vi "Stage 3.3 Placing Process into subVIs.vi"() -> ()   [LabVIEW 2020]
uses:
  HRM-User_events.ctl
  HRM-init_cluster.ctl
panel:
  out "Process Error":errorcluster
  out "error out":errorcluster
  out "raw data":waveform(dbl)
  out "error out Hardware":errorcluster
  in  "Addition signal to remove (0) [s]":dbl
  out "Pulse":dbl
  out "Filtered":waveform(dbl)(graph)
  in  "Samples size (10) [s]":i32=10
  out "unfiltered wf":waveform(dbl)(graph)
  in  "Stop":bool
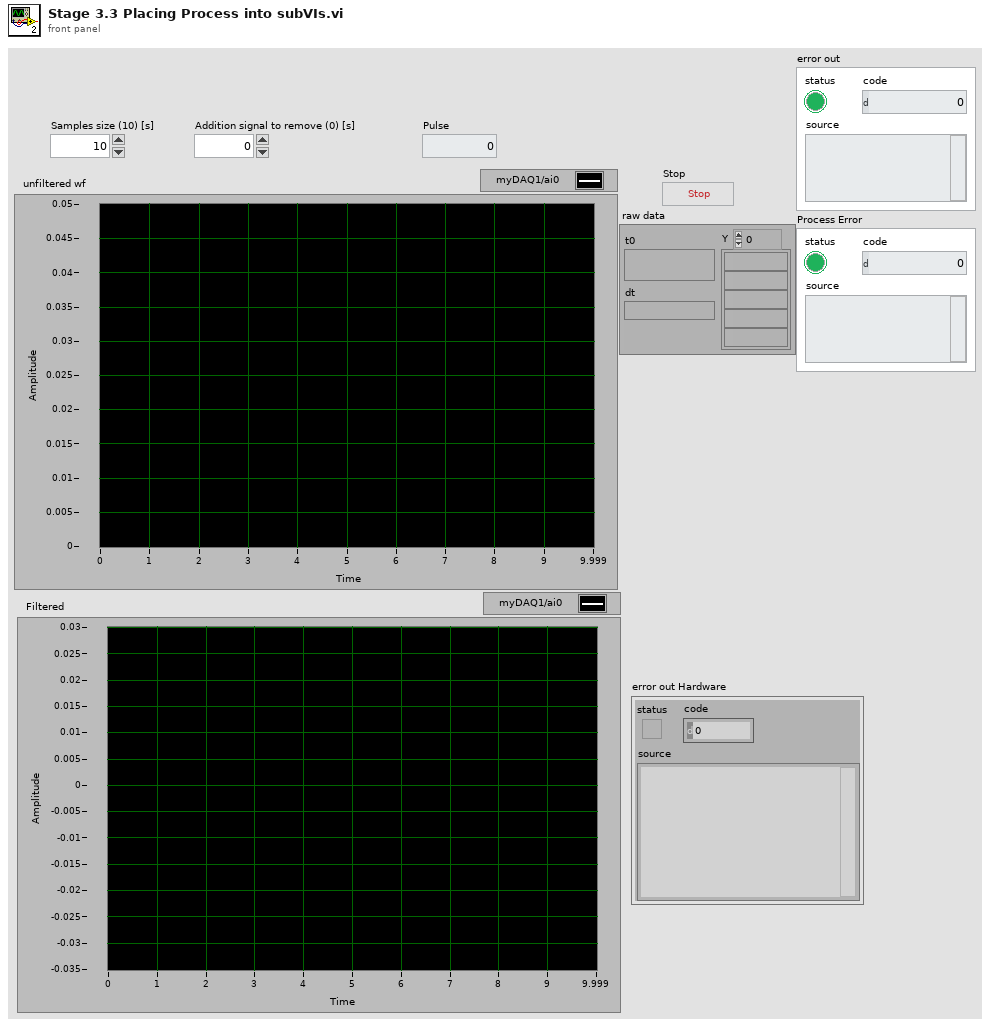
[diagram p1: front panel]
types:
  T1 = typedef "HRM-init_cluster.ctl" = cluster{"User events":T2}
  T2 = typedef "HRM-User_events.ctl" = cluster{"Signal to remove":refnum<user-event>, "Sample size":refnum<user-event>, "Filtered wf":refnum<user-event>, "Unfiltered wf":refnum<user-event>, "Raw wf":refnum<user-event>, "Pulse":refnum<user-event>, "stop":refnum<user-event>}
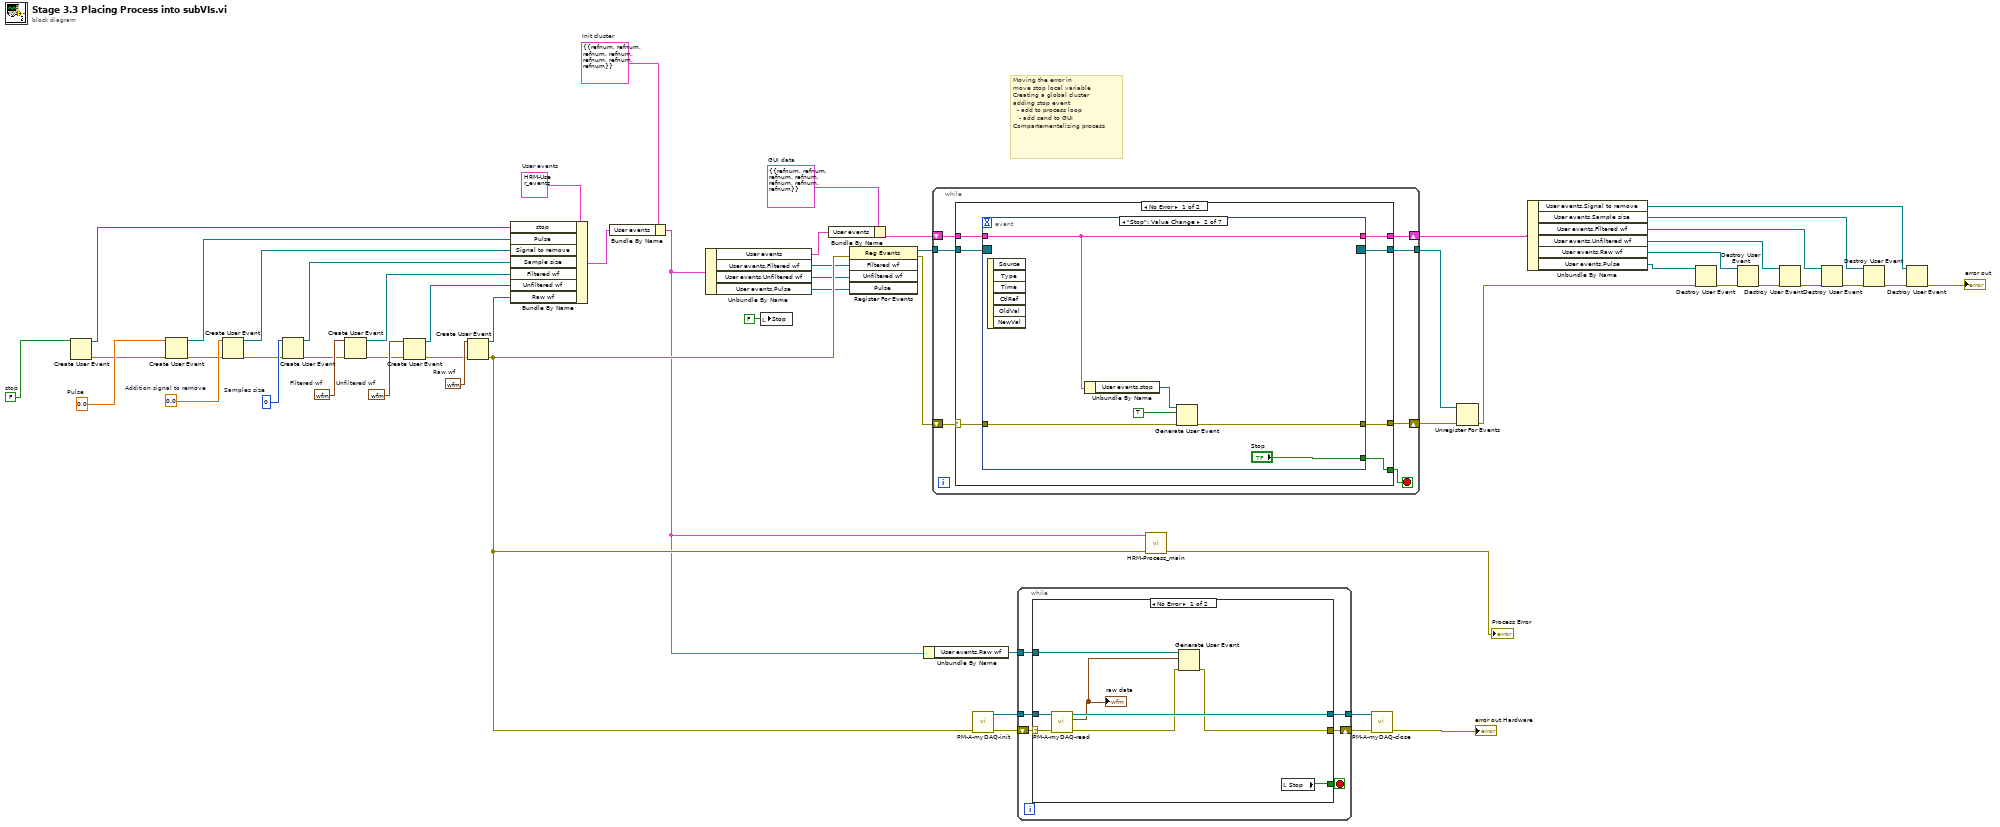
[diagram p0: block diagram]
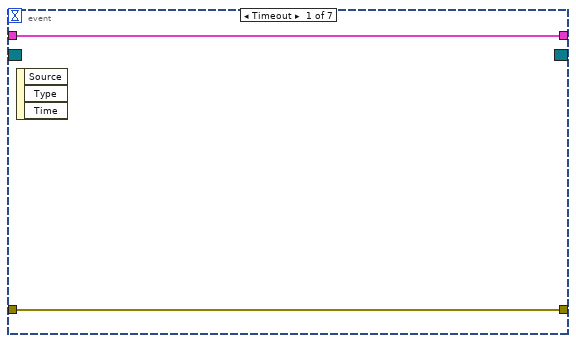
[diagram p2: hidden frame]
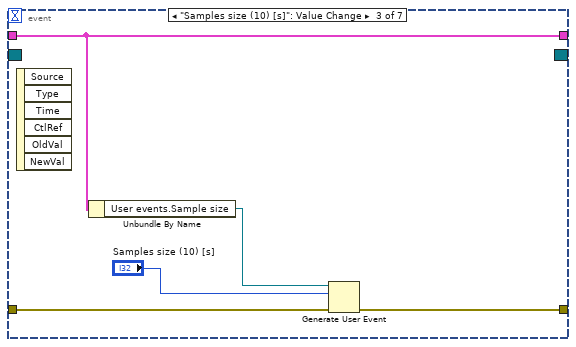
[diagram p3: hidden frame]
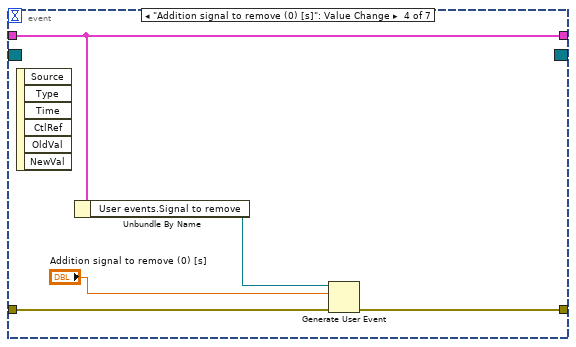
[diagram p4: hidden frame]
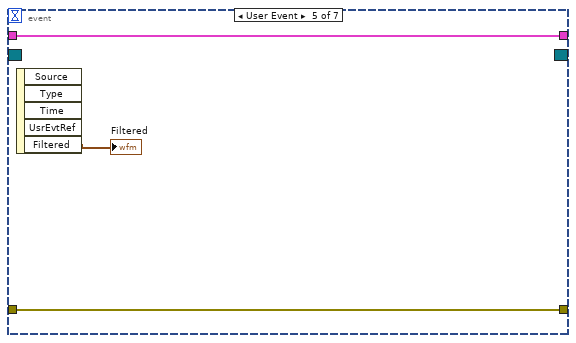
[diagram p5: hidden frame]
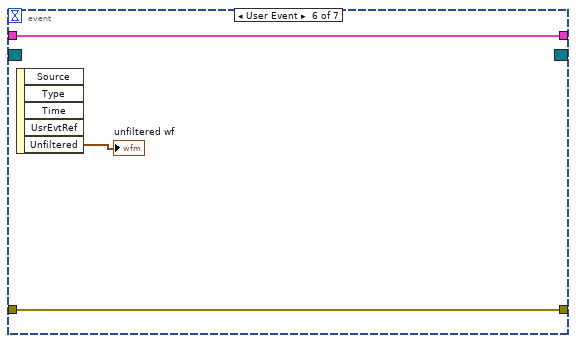
[diagram p6: hidden frame]
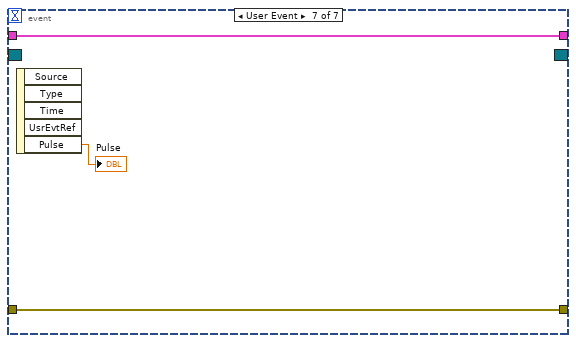
[diagram p7: hidden frame]
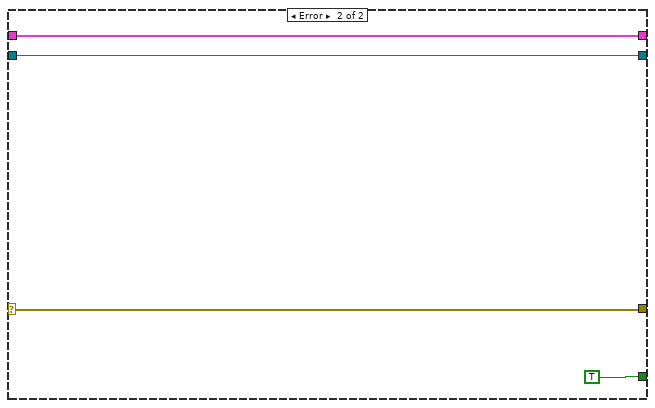
[diagram p8: hidden frame]
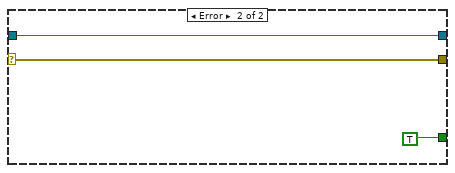
[diagram p9: hidden frame]
diagram:
  w6 = FALSE  # stop
  w13 = T1 {"User events"={"Signal to remove"=refnum, "Sample size"=refnum, "Filtered wf"=refnum, "Unfiltered wf"=refnum, "Raw wf"=refnum, "Pulse"=refnum, "stop"=refnum}}  # Init cluster
  w33 = cluster{"User events":T2} {"User events"={"Signal to remove"=refnum, "Sample size"=refnum, "Filtered wf"=refnum, "Unfiltered wf"=refnum, "Raw wf"=refnum, "Pulse"=refnum, "stop"=refnum}}  # GUI data
  w38 = 0.0  # Pulse
  w45 = T2 {"Signal to remove"=refnum, "Sample size"=refnum, "Filtered wf"=refnum, "Unfiltered wf"=refnum, "Raw wf"=refnum, "Pulse"=refnum, "stop"=refnum}  # User events
  w50 = 0  # Samples size
  w51 = 0.0  # Addition signal to remove
  w52 = waveform(dbl) {"t0"=timestamp(0 s since 1904-01-01), "dt"=1.0, "Y"=[]}  # Filtered wf
  w53 = waveform(dbl) {"t0"=timestamp(0 s since 1904-01-01), "dt"=1.0, "Y"=[]}  # Unfiltered wf
  w54 = waveform(dbl) {"t0"=timestamp(0 s since 1904-01-01), "dt"=1.0, "Y"=[]}  # Raw wf
  # "Moving the error in\nmove stop local variable\nCreating a global cluster\nadding stop event\n  - add to process loop\n   - add send to GUI\nCompartementelizing process"
  n1 = Create User Event(user event datatype=w6) -> (user event=w4:refnum<user-event>, error out=w5:errorcluster)  [unwired: 1 in]
  n2 = Create User Event(user event datatype=w38, error in=w5) -> (user event=w37:refnum<user-event>, error out=w36:errorcluster)
  n3 = Create User Event(user event datatype=w51, error in=w36) -> (user event=w44:refnum<user-event>, error out=w46:errorcluster)
  n4 = Create User Event(user event datatype=w50, error in=w46) -> (user event=w43:refnum<user-event>, error out=w47:errorcluster)
  n5 = Create User Event(user event datatype=w52, error in=w47) -> (user event=w42:refnum<user-event>, error out=w48:errorcluster)
  n6 = Create User Event(user event datatype=w53, error in=w48) -> (user event=w41:refnum<user-event>, error out=w49:errorcluster)
  n7 = Create User Event(user event datatype=w54, error in=w49) -> (user event=w40:refnum<user-event>, error out=w14:errorcluster)
  n8 = Bundle By Name(cluster=w45, "stop"=w4, "Pulse"=w37, "Signal to remove"=w44, "Sample size"=w43, "Filtered wf"=w42, "Unfiltered wf"=w41, "Raw wf"=w40) -> (w12:T2)
  n9 = Bundle By Name(cluster=w13, "User events"=w12) -> (w11:T1)
  n10 = Unbundle By Name(w11) -> ("User events"=w10:T2, "User events.Filtered wf"=w9:refnum<user-event>, "User events.Unfiltered wf"=w8:refnum<user-event>, "User events.Pulse"=w7:refnum<user-event>)
  n11 = local write "Stop"(FALSE ("Stop")) -> ()
  n12 = Bundle By Name(cluster=w33, "User events"=w10) -> (w15:cluster{"User events":T2})
  n13 = register-events(error in=w14, w9, w8, w7) -> (reference out=w35:refnum<event-registration>, error out=w32:errorcluster)  [unwired: 1 in]
  n14 = Unbundle By Name(w11) -> ("User events.Raw wf"=w39:refnum<user-event>)
  n15 = while {
    tunnel: w35 -> [w64]
    shift-right: [w60] -> w30
    shift-left: w32 -> [w61]
    shift-right: [w59] -> w29
    shift-left: w15 -> [w63]
    tunnel: [w58] -> w31
    stop <- w62 stop-if-true
    n16 = case shown="No Error" w61 {
      selector: w61 -> [w68 w101]
      tunnel: [w69 TRUE ("Stop")] -> w62
      tunnel: [w67 w101] -> w60
      tunnel: w64 -> [w71 w99]
      tunnel: w63 -> [w70 w100]
      tunnel: [w66 w100] -> w59
      tunnel: [w65 w99] -> w58
      frame No Error {
        n17 = event shown="[1] \"Stop\": Value Change" {
          selector: w71 -> [_ _ _ _ _ _ _]
          dyn-events: [_ _ _ _ _ _ _] -> w65
          timeout: _ -> [_ _ _ _ _ _ _]
          tunnel: w70 -> [w73 w78 w82 w87 w91 w94 w97]
          tunnel: [_ "Stop" _ _ _ _ _] -> w69
          tunnel: [w72 w75 w83 w88 w92 w95 w98] -> w67
          tunnel: w68 -> [w72 w76 w84 w89 w92 w95 w98]
          tunnel: [w73 w78 w82 w87 w91 w94 w97] -> w66
          event Timeout {
            n18 = event-data() -> ()  [unwired: 1 in, 3 out]
          }
          event "Stop": Value Change {
            n19 = event-data() -> ()  [unwired: 1 in, 6 out]
            n20 = Unbundle By Name(w78) -> ("User events.stop"=w77:refnum<user-event>)
            n21 = Generate User Event(user event=w77, event data cluster=TRUE ("event data"), error in=w76) -> (error out=w75:errorcluster)  [unwired: 1 in, 1 out]
          }
          event "Samples size (10) [s]": Value Change {
            n22 = event-data() -> ()  [unwired: 1 in, 6 out]
            n23 = Unbundle By Name(w82) -> ("User events.Sample size"=w81:refnum<user-event>)
            n24 = Generate User Event(user event=w81, event data cluster="Samples size (10) [s]", error in=w84) -> (error out=w83:errorcluster)  [unwired: 1 in, 1 out]
          }
          event "Addition signal to remove (0) [s]": Value Change {
            n25 = event-data() -> ()  [unwired: 1 in, 6 out]
            n26 = Unbundle By Name(w87) -> ("User events.Signal to remove"=w86:refnum<user-event>)
            n27 = Generate User Event(user event=w86, event data cluster="Addition signal to remove (0) [s]", error in=w89) -> (error out=w88:errorcluster)  [unwired: 1 in, 1 out]
          }
          event User Event {
            n28 = event-data() -> ("Filtered"=→"Filtered":waveform(dbl))  [unwired: 1 in, 4 out]
          }
          event User Event {
            n29 = event-data() -> ("Unfiltered"=→"unfiltered wf":waveform(dbl))  [unwired: 1 in, 4 out]
          }
          event User Event {
            n30 = event-data() -> ("Pulse"=→"Pulse":dbl)  [unwired: 1 in, 4 out]
          }
        }
      }
      frame Error {
      }
    }
  }
  n31 = call "PM-A-myDAQ-init.vi"("error in"=w14) -> ("error out"=w34:errorcluster, "Refnum out"=w55:refnum<k21>)  [unwired: 9 in]
  n32 = while {
    tunnel: w55 -> [w108]
    tunnel: [w106] -> w56
    shift-right: [w105] -> w57
    shift-left: w34 -> [w107]
    tunnel: w39 -> [w103]
    stop <- w104 stop-if-true
    n33 = case shown="No Error" w107 {
      selector: w107 -> [w115 w118]
      tunnel: w108 -> [w116 w117]
      tunnel: [w114 w117] -> w106
      tunnel: [w110 w118] -> w105
      tunnel: [w113 TRUE ("Stop")] -> w104
      tunnel: w103 -> [w109 _]
      frame No Error {
        n34 = call "PM-A-myDAQ-read.vi"("error in (no error)"=w115, "Refnum in"=w116) -> ("error out"=w111:errorcluster, "data"=w112:waveform(dbl), "Refnum out"=w114:refnum<k21>)  [unwired: 7 in]
        "raw data" <- w112
        n35 = Generate User Event(user event=w109, event data cluster=w112, error in=w111) -> (error out=w110:errorcluster)  [unwired: 1 in, 1 out]
        n36 = local read "Stop"() -> (w113:bool)
      }
      frame Error {
      }
    }
  }
  n37 = call "HRM-Process_main.vi"("error in (no error)"=w14, "Init cluster"=w11) -> ("error out"=→"Process Error":errorcluster)  [unwired: 9 in]
  n38 = call "PM-A-myDAQ-close.vi"("error in (no error)"=w57, "Refnum in"=w56) -> ("error out"=→"error out Hardware":errorcluster)  [unwired: 9 in]
  n39 = Unregister For Events(event registration refnum=w31, error in=w30) -> (error out=w17:errorcluster)
  n40 = Unbundle By Name(w29) -> ("User events.Signal to remove"=w18:refnum<user-event>, "User events.Sample size"=w19:refnum<user-event>, "User events.Filtered wf"=w20:refnum<user-event>, "User events.Unfiltered wf"=w21:refnum<user-event>, "User events.Raw wf"=w22:refnum<user-event>, "User events.Pulse"=w23:refnum<user-event>)
  n41 = Destroy User Event(user event=w23, error in=w17) -> (error out=w24:errorcluster)
  n42 = Destroy User Event(user event=w22, error in=w24) -> (error out=w28:errorcluster)
  n43 = Destroy User Event(user event=w21, error in=w28) -> (error out=w27:errorcluster)
  n44 = Destroy User Event(user event=w20, error in=w27) -> (error out=w26:errorcluster)
  n45 = Destroy User Event(user event=w19, error in=w26) -> (error out=w25:errorcluster)
  n46 = Destroy User Event(user event=w18, error in=w25) -> (error out=→"error out":errorcluster)
